vi "Recive_Frame_TO_Form.vi"(7 "TRCount":u32, 9 "CAN_OBJ_RN":T1[](array[typedef]), 10 "T/R":bool, 11 "NUM":i32) -> (2 "TRCount Out":u32, 3 "数组":string[][](array[string]))   [LabVIEW 2020, in "ZLG_CAN.lvlib"]
uses:
  ZLG_CAN.lvlib
  CAN_OBJ_R.ctl
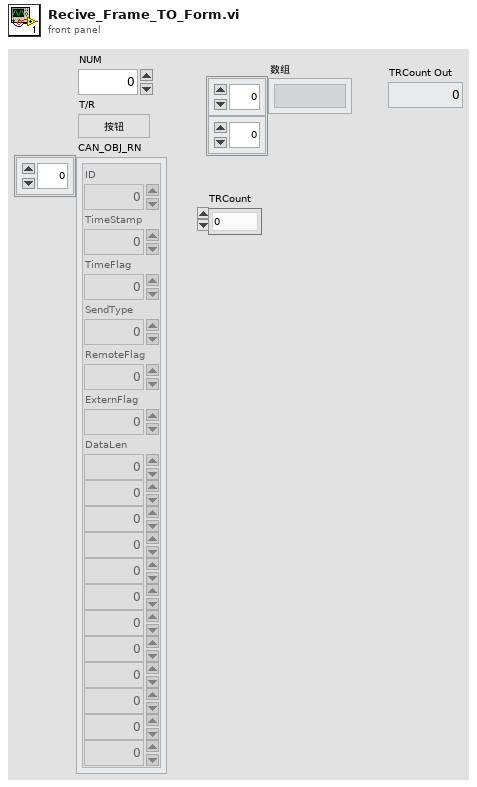
[diagram p1: front panel]
types:
  T1 = typedef "ZLG_CAN.lvlib/CAN_OBJ_R.ctl" = cluster{"ID":u32, "TimeStamp":u32, "TimeFlag":u8, "SendType":u8, "RemoteFlag":u8, "ExternFlag":u8, "DataLen":u8, "数值":u8, "数值":u8, "数值":u8, "数值":u8, "数值":u8, "数值":u8, "数值":u8, "数值":u8, "数值":u8, "数值":u8, "数值":u8}
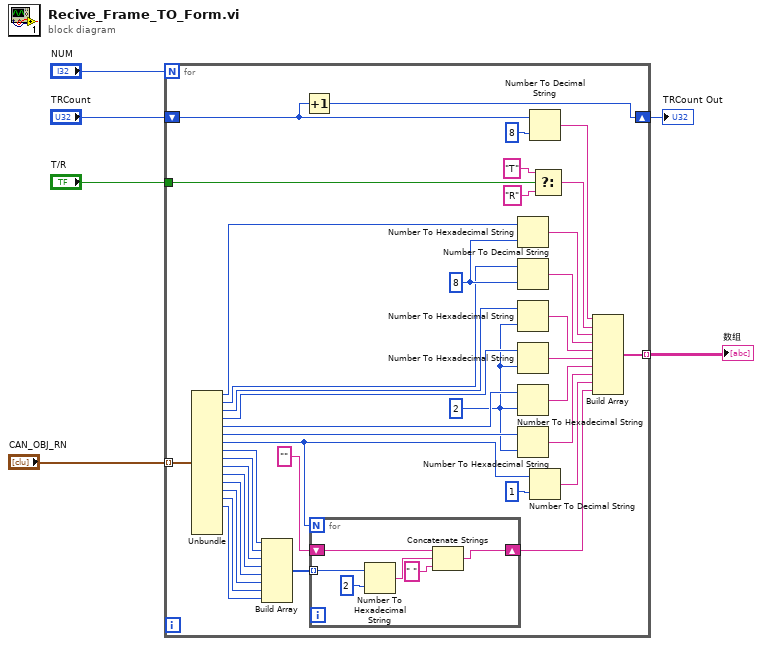
[diagram p0: block diagram]
diagram:
  n1 = for {
    N: "NUM" -> [_]
    tunnel: "CAN_OBJ_RN" -> [w14] mode=indexing
    shift-right: [w10] -> w1
    shift-left: "TRCount" -> [w9]
    tunnel: "T/R" -> [w8]
    tunnel: [w7] -> w3 mode=indexing
    w21 = 2
    w42 = 8
    n2 = Unbundle(w14) -> ("ID"=w44:u32, "TimeStamp"=w41:u32, "TimeFlag"=w22:u8, "SendType"=w39:u8, "RemoteFlag"=w40:u8, "ExternFlag"=w38:u8, "DataLen"=w15:u8, "数值"=w31:u8, "数值"=w30:u8, "数值"=w29:u8, "数值"=w28:u8, "数值"=w27:u8, "数值"=w26:u8, "数值"=w24:u8, "数值"=w25:u8)  [unwired: 3 out]
    n3 = Build Array(w31, w30, w29, w28, w27, w26, w24, w25) -> (w16:u8[])
    n4 = Increment(x=w9) -> (x+1=w10:u32)
    n5 = for {
      N: w15 -> [_]
      shift-right: [w47] -> w18
      shift-left: "" -> [w45]
      tunnel: w16 -> [w46] mode=indexing
      n6 = Number To Hexadecimal String(1:i16 2 ("width (-)"), 2:w46) -> (0:w49:string)
      n7 = Concatenate Strings(w45, w49, " " ("string")) -> (w47:string)
    }
    n8 = Number To Hexadecimal String(1:w42, 2:w44) -> (0:w43:string)
    n9 = Number To Decimal String(number=w41, width (-)=w42) -> (decimal integer string=w37:string)
    n10 = Number To Hexadecimal String(1:w21, 2:w22) -> (0:w23:string)
    n11 = Number To Hexadecimal String(1:w21, 2:w39) -> (0:w36:string)
    n12 = Number To Hexadecimal String(1:w21, 2:w40) -> (0:w35:string)
    n13 = Number To Hexadecimal String(1:w21, 2:w38) -> (0:w34:string)
    n14 = Number To Decimal String(number=w9, width (-)=i16 8) -> (decimal integer string=w19:string)
    n15 = Number To Decimal String(number=w15, width (-)=1) -> (decimal integer string=w32:string)
    n16 = Select(t="T", s=w8, f="R") -> (s? t:f=w12:string)
    n17 = Build Array(w19, w12, w43, w37, w23, w36, w35, w34, w32, w18) -> (w7:string[])
  }
  "数组" <- w3
  "TRCount Out" <- w1
